vi "글꼴설정.vi"() -> ()   [LabVIEW 2014]
uses:
  System.Windows.Forms
  System.Drawing
panel:
  out "Name":string
  out "Size":sgl
  out "에러 출력":errorcluster
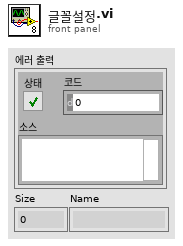
[diagram p1: front panel]
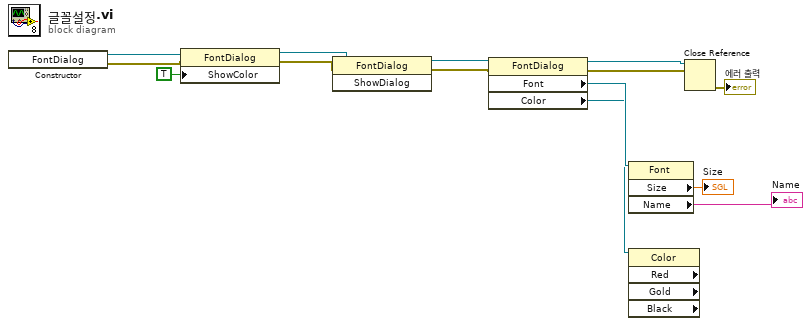
[diagram p0: block diagram]
diagram:
  n1 = constructor class="FontDialog"() -> (reference out=w14:refnum<k24>, error out=w10:errorcluster)  [unwired: 3 in, 1 out]
  n2 = property class="FontDialog"(reference=w14, error in=w10, "ShowColor"=TRUE) -> (reference out=w13:refnum<k24>, error out=w9:errorcluster)
  n3 = invoke class="FontDialog" method="ShowDialog"(reference=w13, error in=w9) -> (reference out=w12:refnum<k24>, error out=w8:errorcluster)  [unwired: 1 in, 1 out]
  n4 = property class="FontDialog"(reference=w12, error in=w8) -> (reference out=w11:refnum<k24>, error out=w7:errorcluster, "Font"=w4:refnum<k24>, "Color"=w3:refnum<k24>)
  n5 = property class="Font"(reference=w4) -> ("Size"=→"Size":sgl, "Name"=→"Name":string)  [unwired: 1 in, 2 out]
  n6 = property class="Color" props=["Red", "Gold", "Black"](reference=w3) -> ()  [unwired: 1 in, 5 out]
  n7 = Close Reference(reference=w11, error in (no error)=w7) -> (error out=→"에러 출력":errorcluster)
